vi "PDFCreator Set Options.vi"(0 "PDFCreator._clsPDFCreator":refnum<k7>, 7 "Options":T1, 11 "error in (no error)":errorcluster) -> (4 "PDFCreator._clsPDFCreator 2":refnum<k7>, 15 "error out":errorcluster)   [LabVIEW 2010]
doc: "Jean-Marc Simard \nJanuary 6, 2010"
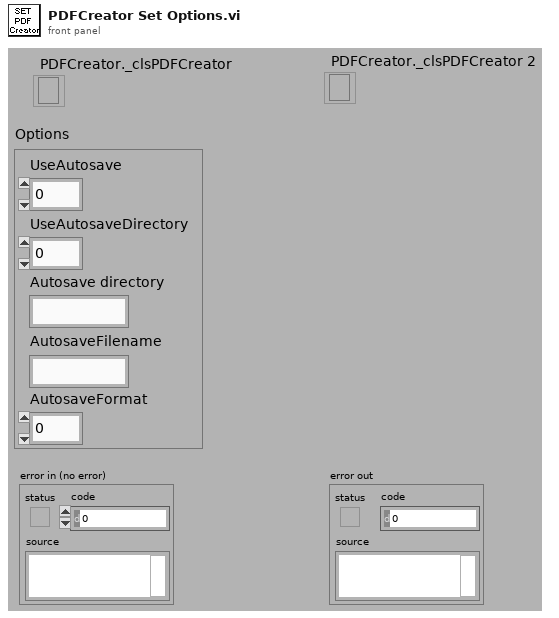
[diagram p1: front panel]
types:
  T1 = cluster{"UseAutosave":i32, "UseAutosaveDirectory":i32, "Autosave directory":string, "AutosaveFilename":string, "AutosaveFormat":i32}
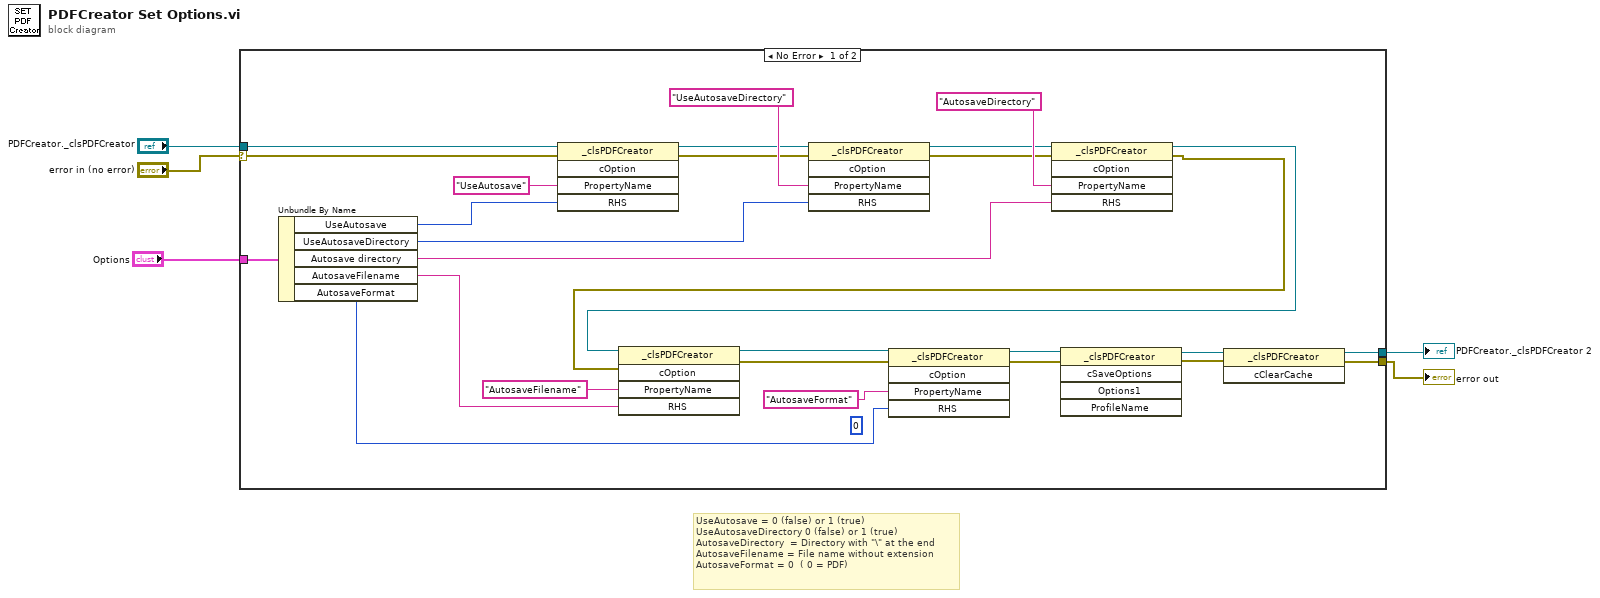
[diagram p0: block diagram]
diagram:
  # "UseAutosave = 0 (false) or 1 (true)\nUseAutosaveDirectory 0 (false) or 1 (true)\nAutosaveDirectory  = Directory with \"\\\" at the end\nAutosaveFilename = File name without extension \nAutosaveFormat = 0  ( 0 = PDF)"
  n1 = case shown="No Error" "error in (no error)" {
    selector: "error in (no error)" -> [w23 w33]
    tunnel: [w22 w34] -> w5
    tunnel: [w21 w33] -> w3
    tunnel: "PDFCreator._clsPDFCreator" -> [w24 w34]
    tunnel: "Options" -> [w20 _]
    frame No Error {
      (unwired) 0
      n2 = Unbundle By Name(w20) -> ("UseAutosave"=w19:i32, "UseAutosaveDirectory"=w16:i32, "Autosave directory"=w14:string, "AutosaveFilename"=w13:string, "AutosaveFormat"=w11:i32)
      n3 = invoke class="_clsPDFCreator" method="cOption"(reference=w24, error in=w23, "PropertyName"="UseAutosave", "RHS"=w19) -> (reference out=w18:refnum<k7>, error out=w17:errorcluster)  [unwired: 1 in, 3 out]
      n4 = invoke class="_clsPDFCreator" method="cOption"(reference=w18, error in=w17, "PropertyName"="UseAutosaveDirectory", "RHS"=w16) -> (reference out=w29:refnum<k7>, error out=w15:errorcluster)  [unwired: 1 in, 3 out]
      n5 = invoke class="_clsPDFCreator" method="cOption"(reference=w29, error in=w15, "PropertyName"="AutosaveDirectory", "RHS"=w14) -> (reference out=w27:refnum<k7>, error out=w8:errorcluster)  [unwired: 1 in, 3 out]
      n6 = invoke class="_clsPDFCreator" method="cOption"(reference=w27, error in=w8, "PropertyName"="AutosaveFilename", "RHS"=w13) -> (reference out=w25:refnum<k7>, error out=w12:errorcluster)  [unwired: 1 in, 3 out]
      n7 = invoke class="_clsPDFCreator" method="cOption"(reference=w25, error in=w12, "PropertyName"="AutosaveFormat", "RHS"=w11) -> (reference out=w10:refnum<k7>, error out=w9:errorcluster)  [unwired: 1 in, 3 out]
      n8 = invoke class="_clsPDFCreator" method="cSaveOptions"(reference=w10, error in=w9) -> (reference out=w7:refnum<k7>, error out=w6:errorcluster)  [unwired: 3 in, 3 out]
      n9 = invoke class="_clsPDFCreator" method="cClearCache"(reference=w7, error in=w6) -> (reference out=w22:refnum<k7>, error out=w21:errorcluster)  [unwired: 1 in, 1 out]
    }
    frame Error {
    }
  }
  "error out" <- w3
  "PDFCreator._clsPDFCreator 2" <- w5
